vi "Disobeying_Graph_ScalesMODCA2.vi"() -> ()   [LabVIEW 2012]
panel:
  out "XScale\nActual\nIncrement":dbl
  out "OK?":bool
  out "YScale Increment":dbl
  out "YScale Max":dbl
  out "YScale Min":dbl
  out "XScale Min":dbl
  out "XScaleMax":dbl
  out "XScale Increment":dbl
  out "rawMS":cluster{dbl[], dbl[]}(graph) caption="Current Mass Spectrum"
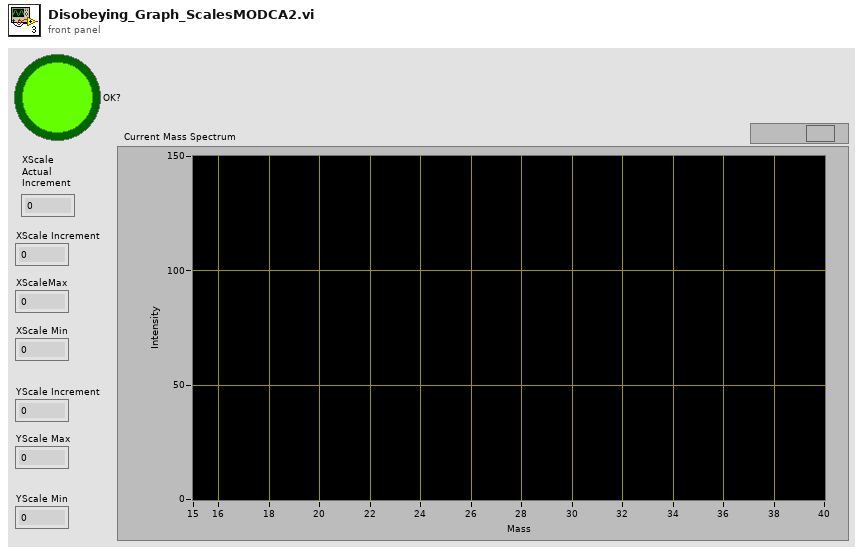
[diagram p1: front panel]
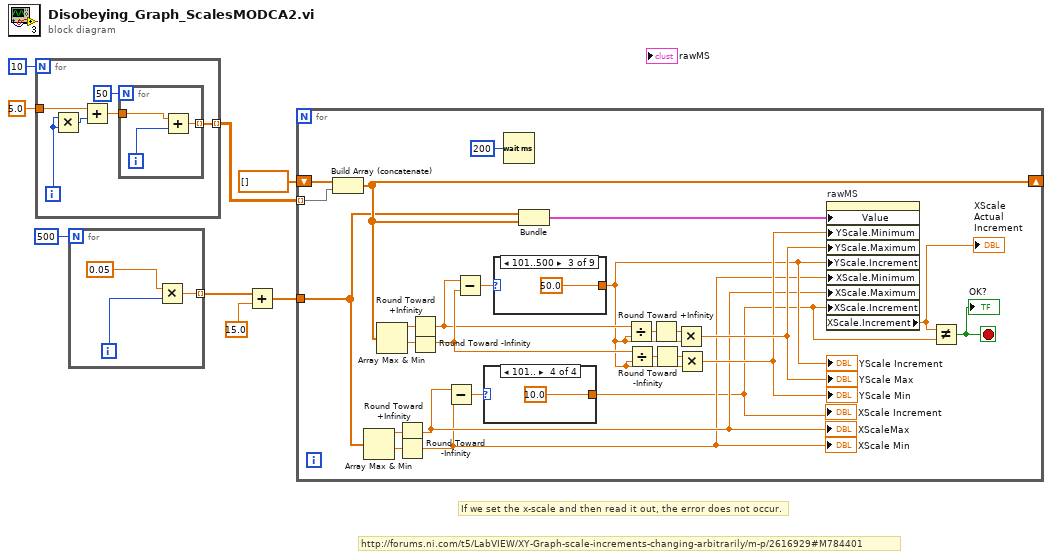
[diagram p0: block diagram]
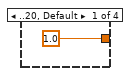
[diagram p2: hidden frame]
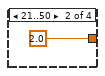
[diagram p3: hidden frame]
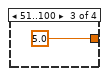
[diagram p4: hidden frame]
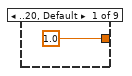
[diagram p5: hidden frame]
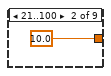
[diagram p6: hidden frame]
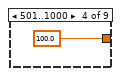
[diagram p7: hidden frame]
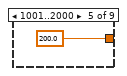
[diagram p8: hidden frame]
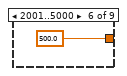
[diagram p9: hidden frame]
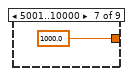
[diagram p10: hidden frame]
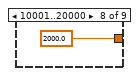
[diagram p11: hidden frame]
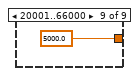
[diagram p12: hidden frame]
diagram:
  # "http://forums.ni.com/t5/LabVIEW/XY-Graph-scale-increments-changing-arbitrarily/m-p/2616929#M784401"
  # "If we set the x-scale and then read it out, the error does not occur."
  n1 = for {
    N: 10 -> [_]
    tunnel: 5.0 -> [w13]
    tunnel: [w11] -> w5 mode=indexing
    i -> [w9]
    n2 = Multiply(x=w9, y=w9) -> (x*y=w10:i32)
    n3 = Add(x=w13, y=w10) -> (x+y=w12:dbl)
    n4 = for {
      N: 50 -> [_]
      tunnel: w12 -> [w17]
      tunnel: [w16] -> w11 mode=indexing
      i -> [w15]
      n5 = Add(x=w17, y=w15) -> (x+y=w16:dbl)
    }
  }
  n6 = for {
    N: 500 -> [_]
    tunnel: [w18] -> w3 mode=indexing
    i -> [w20]
    n7 = Multiply(x=0.05, y=w20) -> (x*y=w18:dbl)
  }
  n8 = Add(x=w3, y=15.0) -> (x+y=w1:dbl[])
  n9 = for {
    tunnel: w1 -> [w27]
    shift-right: [w31] -> _
    shift-left: dbl[] [] -> [w46]
    tunnel: w5 -> [w45] mode=indexing
    stop <- w25 stop-if-true
    n10 = Build Array (concatenate)(w46, w45) -> (w31:dbl[])
    n11 = Array Max & Min(array=w27) -> (max value=w28:dbl, min value=w29:dbl)  [unwired: 2 out]
    n12 = Array Max & Min(array=w31) -> (max value=w35:dbl, min value=w36:dbl)  [unwired: 2 out]
    n13 = Round Toward +Infinity(x=w28) -> (ceil(x): smallest int >= x=w26:dbl)
    "XScaleMax" <- w26
    n14 = Round Toward -Infinity(1:w29) -> (0:w24:dbl)
    "XScale Min" <- w24
    n15 = Round Toward +Infinity(x=w35) -> (ceil(x): smallest int >= x=w40:dbl)
    n16 = Round Toward -Infinity(1:w36) -> (0:w43:dbl)
    n17 = Subtract(x=w26, y=w24) -> (x-y=w30:dbl)
    n18 = Subtract(x=w40, y=w43) -> (x-y=w37:dbl)
    n19 = case shown="101.." w30 {
      tunnel: [1.0 2.0 5.0 10.0] -> w22
      frame ..20, Default {
      }
      frame 21..50 {
      }
      frame 51..100 {
      }
      frame 101.. {
      }
    }
    "XScale Increment" <- w22
    n20 = case shown="101..500" w37 {
      tunnel: [1.0 10.0 50.0 100.0 200.0 500.0 1000.0 2000.0 5000.0] -> w32
      frame ..20, Default {
      }
      frame 21..100 {
      }
      frame 101..500 {
      }
      frame 501..1000 {
      }
      frame 1001..2000 {
      }
      frame 2001..5000 {
      }
      frame 5001..10000 {
      }
      frame 10001..20000 {
      }
      frame 20001..66000 {
      }
    }
    "YScale Increment" <- w32
    n21 = Wait (ms)(milliseconds to wait=u32 200) -> ()  [unwired: 1 out]
    n22 = Bundle(w27, w31) -> (w23:cluster{dbl[], dbl[]})  [unwired: 1 in]
    n23 = Divide(x=w40, y=w32) -> (x/y=w38:dbl)
    n24 = Divide(x=w43, y=w32) -> (x/y=w41:dbl)
    n25 = Round Toward +Infinity(x=w38) -> (ceil(x): smallest int >= x=w39:dbl)
    n26 = Round Toward -Infinity(1:w41) -> (0:w42:dbl)
    n27 = Multiply(x=w39, y=w32) -> (x*y=w34:dbl)
    "YScale Max" <- w34
    n28 = Multiply(x=w42, y=w32) -> (x*y=w33:dbl)
    "YScale Min" <- w33
    n29 = property on="rawMS" class="XYGraph (strict)"("Value"=w23, "YScale.Minimum"=w33, "YScale.Maximum"=w34, "YScale.Increment"=w32, "XScale.Minimum"=w24, "XScale.Maximum"=w26, "XScale.Increment"=w22) -> ("XScale.Increment"=w21:dbl)  [unwired: 2 in, 2 out]
    "XScale\nActual\nIncrement" <- w21
    n30 = Not Equal?(x=w21, y=w22) -> (x != y?=w25:bool)
    "OK?" <- w25
  }
